vi "Insert with table create.vi"(6 "Data variant":variant, 7 "Max string size(60)":i32=30, 8 "error in":errorcluster, 9 "Table Columns":string[](array[string]), 10 "Table In":string, 11 "connection ref IN":T1) -> (0 "error out":errorcluster, 3 "connection reference out":T1)   [LabVIEW 2009, in "Database Lib.lvlib"]
doc: "Creates a table if one does not exist.\nInserts a record into the table."
uses:
  Database Lib.lvlib
  <vilib>/addons/database/Connection.llb/Conn ObjectReference.ctl
  <vilib>/addons/database/NI_Database_API.lvlib
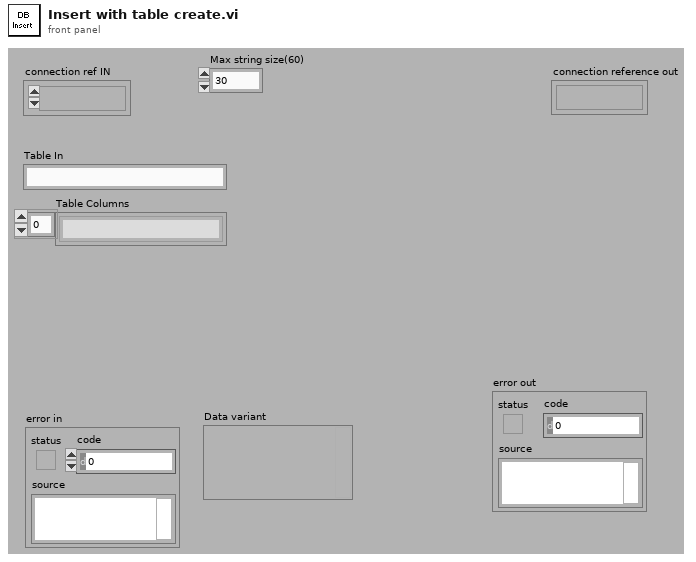
[diagram p1: front panel]
types:
  T1 = typedef "NI_Database_API.lvlib/Conn ObjectReference.ctl" = refnum<k1>
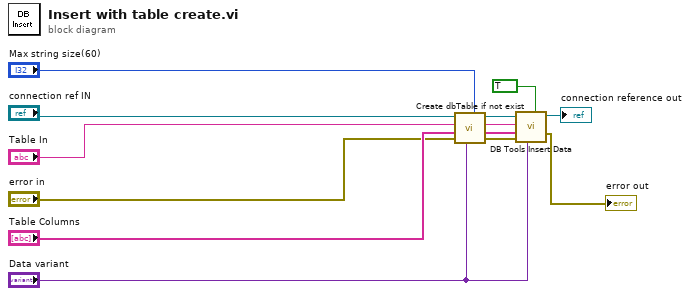
[diagram p0: block diagram]
diagram:
  n1 = call "Create dbTable if not exist.vi"("Max string size(30)"="Max string size(60)", "data"="Data variant", "error in (no error)"="error in", "columns"="Table Columns", "table name"="Table In", "connection reference"="connection ref IN") -> ("error out"=w3:errorcluster, "columns out"=w4:string[], "table name out"=w5:string, "connection reference out"=w6:T1)  [unwired: 1 in, 1 out]
  n2 = call <vilib>:"DB Tools Insert Data.vi"("create table? (f)"=TRUE, "data"="Data variant", "error in (no error)"=w3, "columns"=w4, "table"=w5, "connection reference"=w6) -> ("error out"=→"error out":errorcluster, "connection reference out"=→"connection reference out":T1)  [unwired: 1 in, 3 out]
